vi "InfoCommand.vi"(8 "PAR":string(combo)="BDNAME", 9 "Parameters list":string[](array[string]), 10 "Board parameter? (F)":bool, 11 "Device Family":T1) -> (2 "info_commands":string[](array[string]), 3 "info_response":string)   [LabVIEW 2020, in "CAEN PSM.lvlib"]
uses:
  CAEN PSM.lvlib
  DeviceFamily.ctl
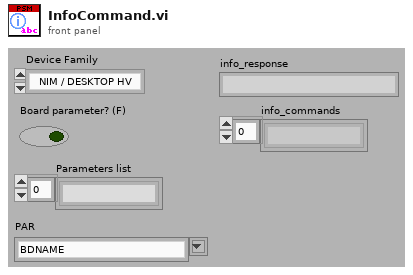
[diagram p1: front panel]
types:
  T1 = typedef "CAEN PSM.lvlib/DeviceFamily.ctl" = enum8{"NIM / DESKTOP HV", "DT55XXE HV", "SMART HV"}
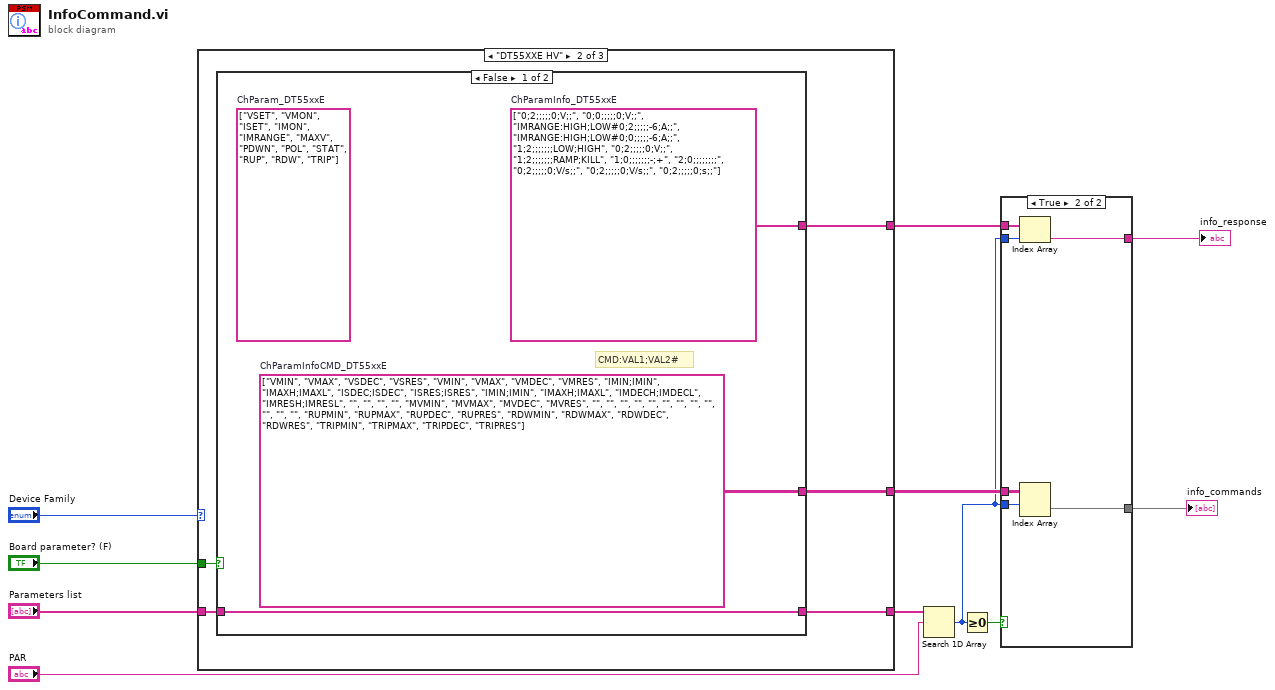
[diagram p0: block diagram]
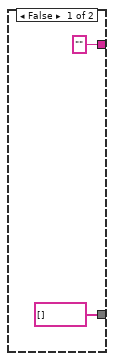
[diagram p2: hidden frame]
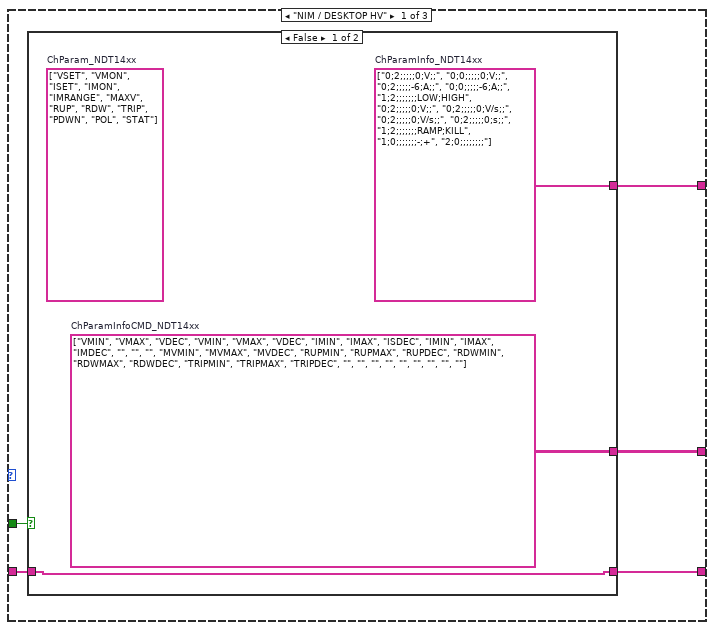
[diagram p3: hidden frame]
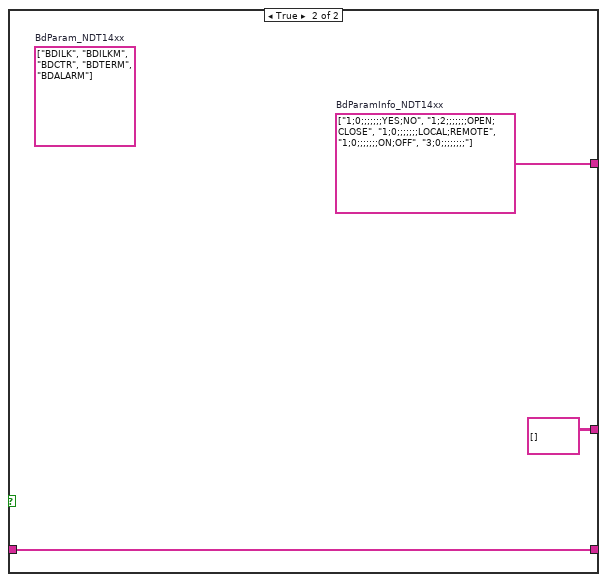
[diagram p4: hidden frame]
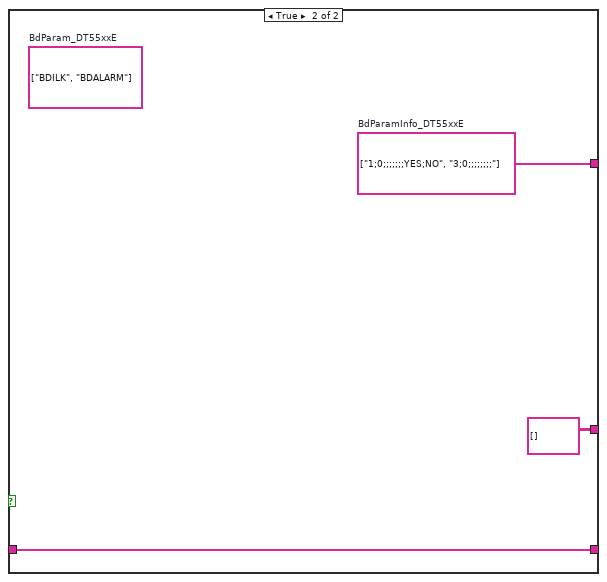
[diagram p5: hidden frame]
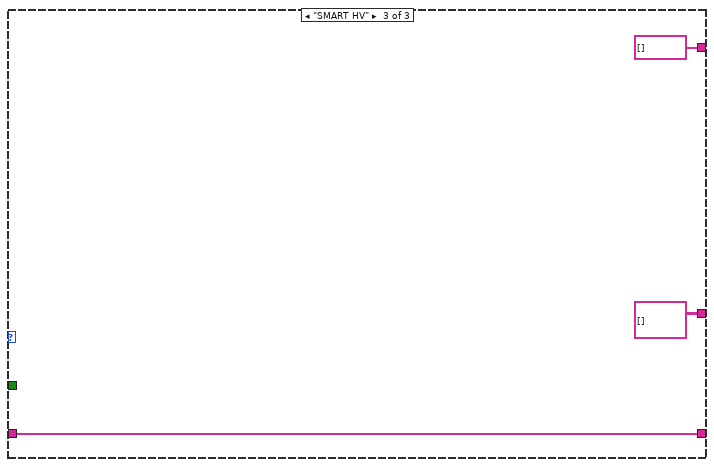
[diagram p6: hidden frame]
diagram:
  n1 = case shown="\"DT55XXE HV\"" "Device Family" {
    tunnel: "Board parameter? (F)" -> [w16 w27 _]
    tunnel: [w14 w26 string[] [] ("BdParamInfo_DT55xxE")] -> w6
    tunnel: [w15 w25 w34] -> w9
    tunnel: [w13 w24 string[][] [] ("ChParamInfoCMD_DT55xxE")] -> w4
    tunnel: "Parameters list" -> [w12 w23 w34]
    frame "NIM / DESKTOP HV" {
      n2 = case shown="False" w16 {
        tunnel: [w17 w20] -> w15
        tunnel: [w19 w22] -> w14
        tunnel: [w18 string[][] [] ("ChParamInfoCMD_NDT14xx")] -> w13
        tunnel: w12 -> [w17 w20]
        frame False {
          w18 = string[][] [["VMIN", "VMAX", "VDEC"], ["VMIN", "VMAX", "VDEC"], ["IMIN", "IMAX", "ISDEC"], ["IMIN", "IMAX", "IMDEC"], ["", "", ""], ["MVMIN", "MVMAX", "MVDEC"], ["RUPMIN", "RUPMAX", "RUPDEC"], ["RDWMIN", "RDWMAX", "RDWDEC"], ["TRIPMIN", "TRIPMAX", "TRIPDEC"], ["", "", ""], ["", "", ""], ["", "", ""]]  # ChParamInfoCMD_NDT14xx
          w19 = string[] ["0;2;;;;;0;V;;", "0;0;;;;;0;V;;", "0;2;;;;;-6;A;;", "0;0;;;;;-6;A;;", "1;2;;;;;;;LOW;HIGH", "0;2;;;;;0;V;;", "0;2;;;;;0;V/s;;", "0;2;;;;;0;V/s;;", "0;2;;;;;0;s;;", "1;2;;;;;;;RAMP;KILL", "1;0;;;;;;;-;+", "2;0;;;;;;;;"]  # ChParamInfo_NDT14xx
          (unwired) string[] ["VSET", "VMON", "ISET", "IMON", "IMRANGE", "MAXV", "RUP", "RDW", "TRIP", "PDWN", "POL", "STAT"]  # ChParam_NDT14xx
        }
        frame True {
          w22 = string[] ["1;0;;;;;;;YES;NO", "1;2;;;;;;;OPEN; CLOSE", "1;0;;;;;;;LOCAL;REMOTE", "1;0;;;;;;;ON;OFF", "3;0;;;;;;;;"]  # BdParamInfo_NDT14xx
          (unwired) string[] ["BDILK", "BDILKM", "BDCTR", "BDTERM", "BDALARM"]  # BdParam_NDT14xx
        }
      }
    }
    frame "DT55XXE HV" {
      n3 = case shown="False" w27 {
        tunnel: [w28 w31] -> w25
        tunnel: [w30 w33] -> w26
        tunnel: [w29 string[][] [] ("ChParamInfoCMD_DT55xxE")] -> w24
        tunnel: w23 -> [w28 w31]
        frame False {
          w29 = string[][] [["VMIN", "VMAX", "VSDEC", "VSRES"], ["VMIN", "VMAX", "VMDEC", "VMRES"], ["IMIN;IMIN", "IMAXH;IMAXL", "ISDEC;ISDEC", "ISRES;ISRES"], ["IMIN;IMIN", "IMAXH;IMAXL", "IMDECH;IMDECL", "IMRESH;IMRESL"], ["", "", "", ""], ["MVMIN", "MVMAX", "MVDEC", "MVRES"], ["", "", "", ""], ["", "", "", ""], ["", "", "", ""], ["RUPMIN", "RUPMAX", "RUPDEC", "RUPRES"], ["RDWMIN", "RDWMAX", "RDWDEC", "RDWRES"], ["TRIPMIN", "TRIPMAX", "TRIPDEC", "TRIPRES"]]  # ChParamInfoCMD_DT55xxE
          w30 = string[] ["0;2;;;;;0;V;;", "0;0;;;;;0;V;;", "IMRANGE:HIGH;LOW#0;2;;;;;-6;A;;", "IMRANGE:HIGH;LOW#0;0;;;;;-6;A;;", "1;2;;;;;;;LOW;HIGH", "0;2;;;;;0;V;;", "1;2;;;;;;;RAMP;KILL", "1;0;;;;;;;-;+", "2;0;;;;;;;;", "0;2;;;;;0;V/s;;", "0;2;;;;;0;V/s;;", "0;2;;;;;0;s;;"]  # ChParamInfo_DT55xxE
          (unwired) string[] ["VSET", "VMON", "ISET", "IMON", "IMRANGE", "MAXV", "PDWN", "POL", "STAT", "RUP", "RDW", "TRIP"]  # ChParam_DT55xxE
          # "CMD:VAL1;VAL2#"
        }
        frame True {
          w33 = string[] ["1;0;;;;;;;YES;NO", "3;0;;;;;;;;"]  # BdParamInfo_DT55xxE
          (unwired) string[] ["BDILK", "BDALARM"]  # BdParam_DT55xxE
        }
      }
    }
    frame "SMART HV" {
    }
  }
  n4 = Search 1D Array(1D array=w9, element="PAR") -> (index of element=w3:i32)  [unwired: 1 in]
  n5 = Greater Or Equal To 0?(x=w3) -> (x >= 0?=w7:bool)
  n6 = case shown="True" w7 {
    tunnel: w6 -> [_ w44]
    tunnel: w3 -> [_ w43]
    tunnel: ["" w42] -> w5
    tunnel: w4 -> [_ w41]
    tunnel: w3 -> [_ w40]
    tunnel: [string[] [] ("ChParamInfoCMD_DT55xxE") w39] -> w2
    frame False {
    }
    frame True {
      n7 = Index Array(array=w44, index=w43) -> (element=w42:string)
      n8 = Index Array(array=w41, index (row)=w40) -> (element=w39:string[])  [unwired: 1 in]
    }
  }
  "info_response" <- w5
  "info_commands" <- w2
